vi "falcon_counts_to_mps.vi"(11 "Velocity (Counts/100ms)":i32) -> (3 "Velocity (m/s)":dbl)   [LabVIEW 2020]
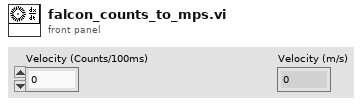
[diagram p1: front panel]
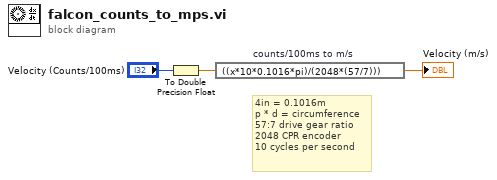
[diagram p0: block diagram]
diagram:
  # "4in = 0.1016m\np * d = circumference\n57:7 drive gear ratio\n2048 CPR encoder\n10 cycles per second"
  n1 = To Double Precision Float(number="Velocity (Counts/100ms)") -> (double precision float=w2:dbl)
  n2 = expression code="((x*10*0.1016*pi)/(2048*(57/7)))" "counts/100ms to m/s"(w2) -> (→"Velocity (m/s)":dbl)
